vi "ERD_Read_List_Builder.vi"(0 "Array":T3(array[cluster]) {"ERD Number" format="%.0x"}, 5 "Error In":errorcluster) -> (14 "Read ERD List":T1[](array[typedef]) {"ERD Number" format="%.0x"}, 19 "Error Out":errorcluster)   [LabVIEW 2016]
doc: "This VI takes an array of ERD Cluster Data. Cluster conatins a boolean to Read the ERD or not, ERD number, name, and data type. It the compiles an array of ERD data to use in ERD Read VI."
uses:
  Common/LabVIEW GEA2 Toolkit/LabVIEW_GEA2_Toolkit.lvlibp/type defs/ERD Read Data In.ctl
  Common/LabVIEW GEA2 Toolkit/LabVIEW_GEA2_Toolkit.lvlibp/type defs/Data Type.ctl
  Common/LabVIEW GEA2 Toolkit/LabVIEW_GEA2_Toolkit.lvlibp
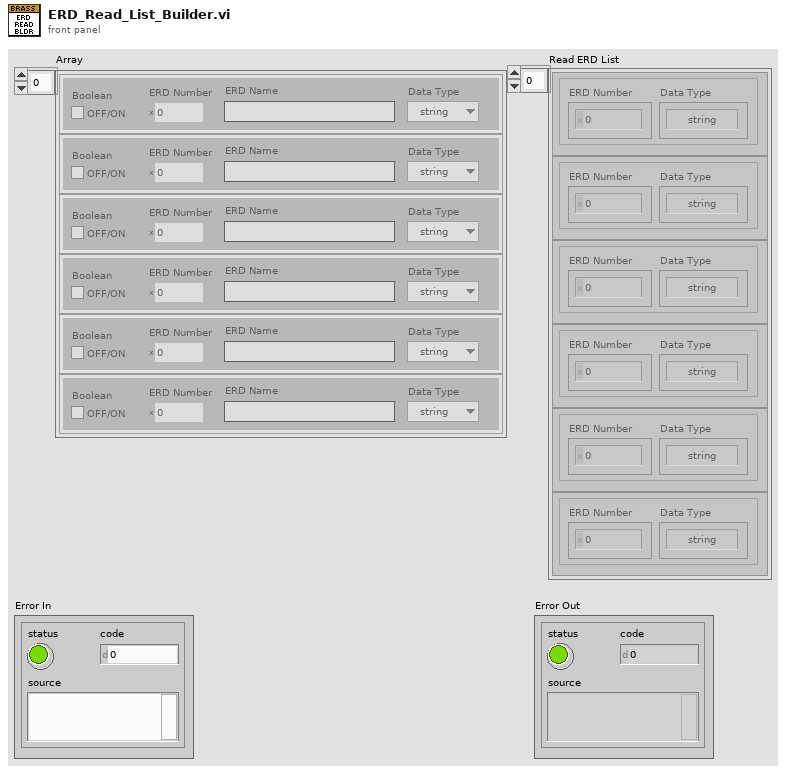
[diagram p1: front panel]
types:
  T1 = typedef "LabVIEW_GEA2_Toolkit.lvlibp/ERD Read Data In.ctl" = cluster{"ERD Number":u16, "Data Type":T2}
  T2 = typedef "LabVIEW_GEA2_Toolkit.lvlibp/Data Type.ctl" = enum16{"string", "boolean", "uint8_t", "uint16_t", "uint32_t", "uint64_t", "int8_t", "int16_t", "int32_t", "int64_t"}
  T3 = cluster{"Boolean":bool, "ERD Number":u16, "ERD Name":string, "Data Type":enum16{"string", "boolean", "uint8_t", "uint16_t", "uint32_t", "uint64_t"}}[]
  T4 = enum16{"string", "boolean", "uint8_t", "uint16_t", "uint32_t", "uint64_t"}
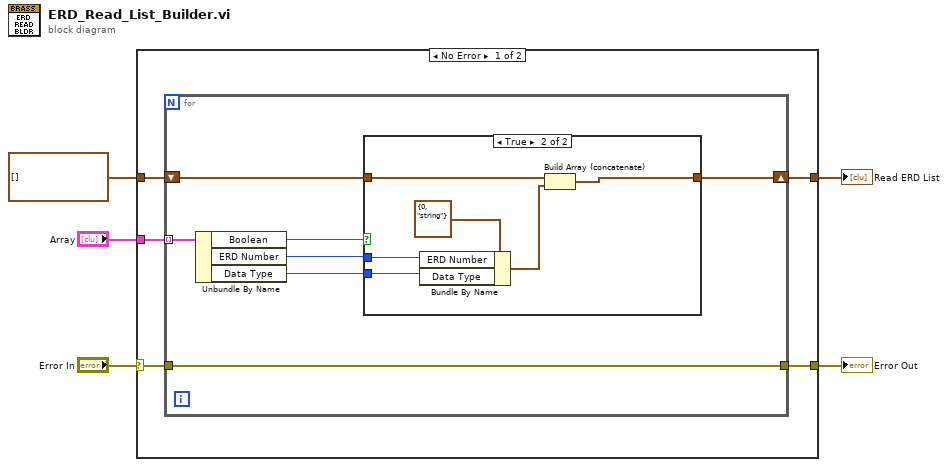
[diagram p0: block diagram]
diagram:
  n1 = case shown="No Error" "Error In" {
    selector: "Error In" -> [w7 w25]
    tunnel: "Array" -> [w10 _]
    tunnel: [w9 _] -> w4
    tunnel: T1[] [] -> [w8 _]
    tunnel: [w6 w25] -> w1
    frame No Error {
      n2 = for {
        tunnel: w10 -> [w17] mode=indexing
        shift-right: [w13] -> w9
        shift-left: w8 -> [w14]
        tunnel: w7 -> [w11]
        tunnel: [w11] -> w6
        n3 = Unbundle By Name(w17) -> ("Boolean"=w16:bool, "ERD Number"=w15:u16, "Data Type"=w12:T4)
        n4 = case shown="True" w16 {
          tunnel: w15 -> [_ w19]
          tunnel: w14 -> [w18 w24]
          tunnel: [w18 w22] -> w13
          tunnel: w12 -> [_ w20]
          frame False {
          }
          frame True {
            n5 = Bundle By Name(cluster=T1 {"ERD Number"=0, "Data Type"=enum."string"} ("ERD Read Data In"), "ERD Number"=w19, "Data Type"=w20) -> (w23:T1)
            n6 = Build Array (concatenate)(w24, w23) -> (w22:T1[])
          }
        }
      }
    }
    frame Error {
    }
  }
  "Read ERD List" <- w4
  "Error Out" <- w1
